vi "Set Gif data.vi"(8 "error in (no error)":errorcluster caption="错误输入（无错误）", 10 "Gif data":string, 11 "Gif Image输入":refnum<class "Gif Image.lvclass">) -> (0 "error out":errorcluster caption="错误输出", 3 "Gif Image输出":refnum<class "Gif Image.lvclass">)   [LabVIEW 2011, in "Gif Image.lvclass"]
uses:
  Gif Image.lvclass
  Gif Image.lvclass/Gif Image.ctl
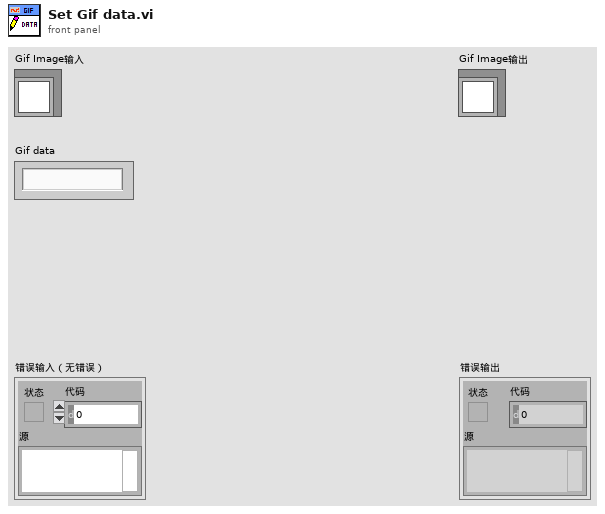
[diagram p1: front panel]
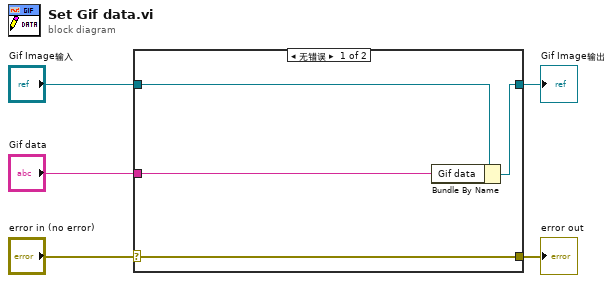
[diagram p0: block diagram]
diagram:
  n1 = case shown="无错误" "error in (no error)" {
    selector: "error in (no error)" -> [w9 w10]
    tunnel: [w9 w10] -> w4
    tunnel: [w7 w11] -> w2
    tunnel: "Gif Image输入" -> [w8 w11]
    tunnel: "Gif data" -> [w6 _]
    frame No Error {
      n2 = Bundle By Name(cluster=w8, "Gif data"=w6) -> (w7:refnum<class "Gif Image.lvclass">)
    }
    frame Error {
    }
  }
  "error out" <- w4
  "Gif Image输出" <- w2
